vi "kvCanObjBufSetFilter.vi"(0 "Object Handle":i32, 1 "Filter Code":u32, 2 "Filter Mask":u32, 3 "error in (no error)":errorcluster, 4 "Channel Handle (input only)":i32) -> (5 "Channel Handle (output only)":i32, 6 "error out":errorcluster)   [LabVIEW 2022 SP3]
doc: "Sets the filter code and mask used to determine when an Automatic Response object buffer should respond."
uses:
  canlib32.dll
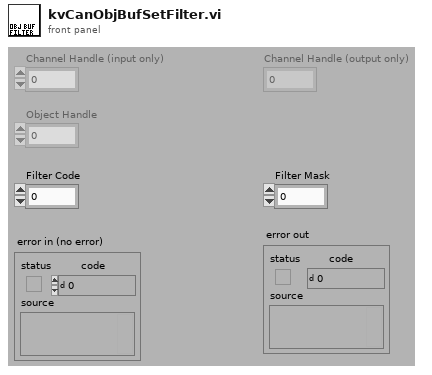
[diagram p1: front panel]
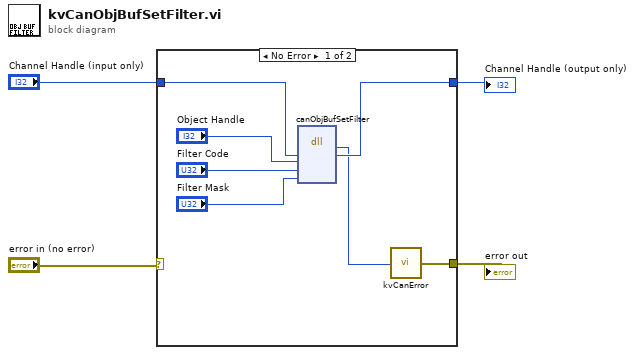
[diagram p0: block diagram]
diagram:
  n1 = case shown="No Error" "error in (no error)" {
    selector: "error in (no error)" -> [_ w13]
    tunnel: [w11 w13] -> w3
    tunnel: "Channel Handle (input only)" -> [w10 w12]
    tunnel: [w9 w12] -> w1
    frame No Error {
      n2 = dll-call lib="canlib32.dll" fn="canObjBufSetFilter"("channelHandle"=w10, "objectBuffer"="Object Handle", "filterCode"="Filter Code", "filterMask"="Filter Mask") -> (w8:i32, "channelHandle"=w9:i32)  [unwired: 6 in, 2 out]
      n3 = call "kvCanError.vi"("error code"=w8) -> ("error out"=w11:errorcluster)
    }
    frame Error {
    }
  }
  "Channel Handle (output only)" <- w1
  "error out" <- w3
